vi "Conductance Background.vi"() -> ()   [LabVIEW 2021]
uses:
  <vilib>/Analysis/NI_AALPro.lvlib
  <vilib>/Analysis/polynomials.llb/1D Polynomial Evaluation (DBL).vi
panel:
  in  "Fit":bool
  in  "polynomial order":i32=2
  in  "BG polynom":dbl[](array[numeric])
  in  "BG2 length":i32
  in  "BG2 start":i32
  in  "BG1 length":i32
  in  "BG1 start":i32
  out "Background":cluster{dbl[], dbl[]}[](graph)
  out "Array - String":string[](array[string])
  out "Temperature vs scan number":cluster{dbl[], dbl[]}(graph)
  in  "Bacground correction":dbl
  in  "Temperature":string="Cryo-Con 32 (12) A"
  in  "Y":string="dIdV"
  in  "X":string="V"
  out "Scans":cluster{dbl[], dbl[]}[](graph)
  out "Scan temperatures":dbl[](array[numeric])
  in  "Scan indexes":i32[](array[numeric])=[1]
  in  "File Path":path=path "C:/Data/m010_072922.tdms"
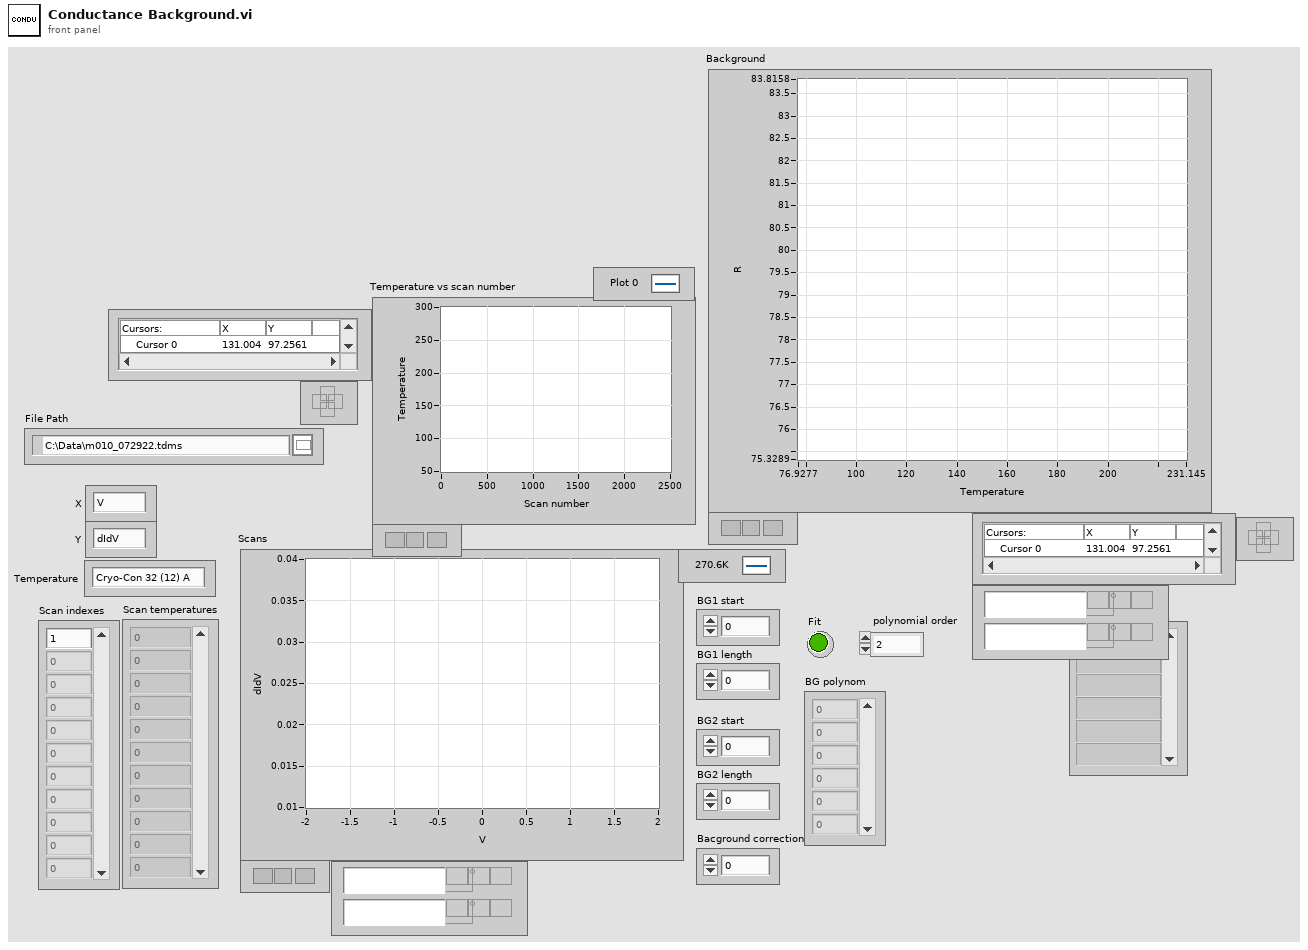
[diagram p1: front panel]
types:
  T1 = enum16{"open", "open or create", "create or replace", "create", "open (read-only)"}
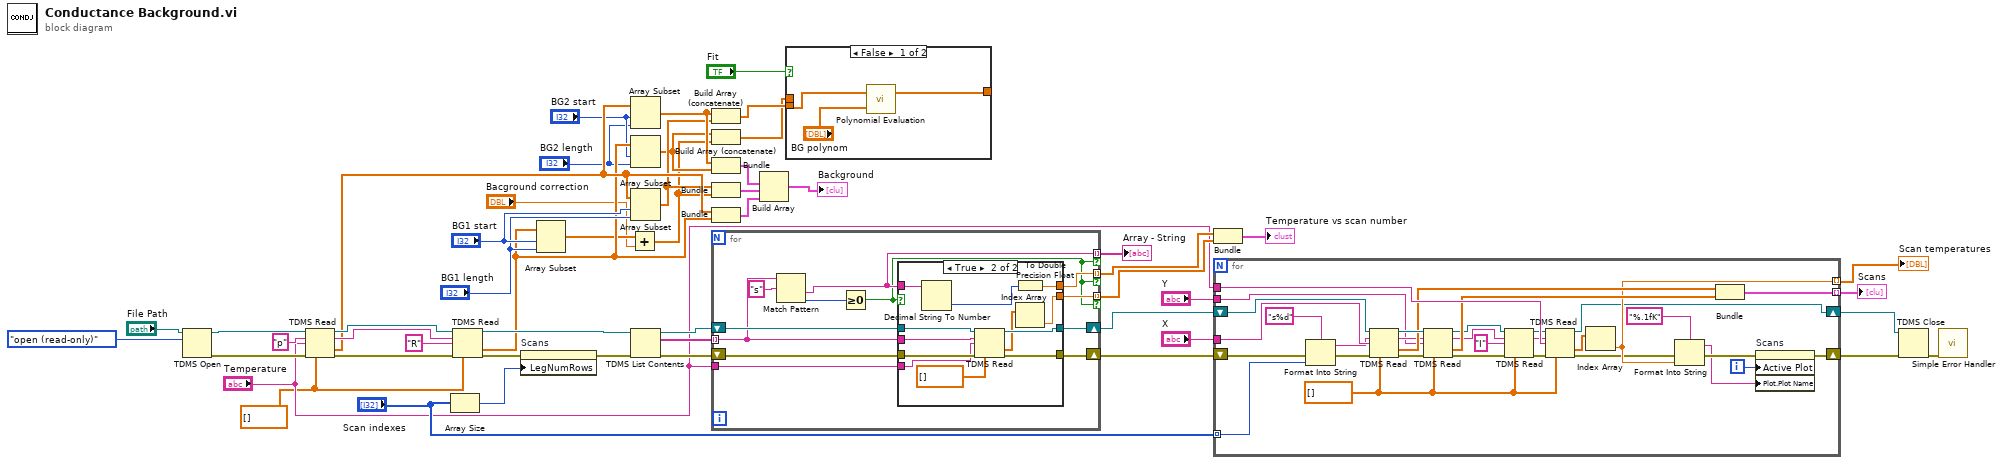
[diagram p0: block diagram]
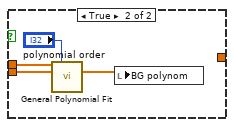
[diagram p2: hidden frame]
diagram:
  w20 = dbl[] []
  n1 = TDMS Open(10:T1."open (read-only)" ("operation (0:open)"), 11:"File Path") -> (0:w42:errorcluster, 3:w28:refnum<k34>)  [unwired: 5 in]
  n2 = TDMS Read(0:w28, 5:"p" ("group name in"), 7:"Temperature", 11:w42, 12:w20) -> (4:w26:refnum<k34>, 6:w23:string, 10:w14:dbl[], 15:w29:errorcluster)  [unwired: 3 in, 2 out]
  n3 = Array Size(array="Scan indexes") -> (size(s)=w43:i32)
  n4 = TDMS Read(0:w26, 5:w23, 7:"R" ("channel name(s) in"), 11:w29, 12:w20) -> (4:w25:refnum<k34>, 10:w13:dbl[], 15:w27:errorcluster)  [unwired: 3 in, 3 out]
  n5 = property on="Scans" class="XYGraph (strict)"(error in=w27, "LegNumRows"=w43) -> (error out=w36:errorcluster)  [unwired: 1 in, 1 out]
  n6 = Array Subset(array=w13, index="BG1 start", length="BG1 length") -> (w9:dbl[])
  n7 = Add(x=w9, y="Bacground correction") -> (x+y=w2:dbl[])
  n8 = Array Subset(array=w14, index="BG2 start", length="BG2 length") -> (w7:dbl[])
  n9 = Array Subset(array=w13, index="BG2 start", length="BG2 length") -> (w3:dbl[])
  n10 = Array Subset(array=w14, index="BG1 start", length="BG1 length") -> (w6:dbl[])
  n11 = TDMS List Contents(4:w36, 7:w25) -> (0:w38:errorcluster, 2:w39:string[], 3:w37:refnum<k34>)  [unwired: 1 in, 1 out]
  n12 = Build Array (concatenate)(w7, w6) -> (w5:dbl[])
  n13 = Build Array (concatenate)(w3, w2) -> (w4:dbl[])
  n14 = Bundle(w7, w3) -> (w12:cluster{dbl[], dbl[]})  [unwired: 1 in]
  n15 = Bundle(w6, w2) -> (w16:cluster{dbl[], dbl[]})  [unwired: 1 in]
  n16 = Bundle(w14, w13) -> (w15:cluster{dbl[], dbl[]})  [unwired: 1 in]
  n17 = for {
    tunnel: w39 -> [w59] mode=indexing
    tunnel: [w54] -> w33 mode=indexing if=w52
    shift-right: [w57] -> w34
    shift-left: w37 -> [w61]
    shift-right: [w56] -> w35
    shift-left: w38 -> [w60]
    tunnel: "Temperature" -> [w58]
    tunnel: [w55] -> w30 mode=indexing if=w52
    tunnel: [w53] -> w31 mode=indexing if=w52
    n18 = Match Pattern(string=w59, regular expression="s") -> (after substring=w54:string, offset past match=w62:i32)  [unwired: 1 in, 2 out]
    n19 = Greater Or Equal To 0?(x=w62) -> (x >= 0?=w52:bool)
    n20 = case shown="True" w52 {
      tunnel: w61 -> [w65 w77]
      tunnel: w60 -> [w64 w76]
      tunnel: w59 -> [_ w74]
      tunnel: w58 -> [_ w73]
      tunnel: [w65 w72] -> w57
      tunnel: [w64 w71] -> w56
      tunnel: [_ w69] -> w55
      tunnel: w54 -> [_ w68]
      tunnel: [_ w66] -> w53
      frame False {
      }
      frame True {
        n21 = Decimal String To Number(string=w68) -> (number=w67:i32)  [unwired: 2 in, 1 out]
        n22 = TDMS Read(0:w77, 5:w74, 7:w73, 11:w76, 12:dbl[] []) -> (4:w72:refnum<k34>, 10:w70:dbl[], 15:w71:errorcluster)  [unwired: 3 in, 3 out]
        n23 = To Double Precision Float(number=w67) -> (double precision float=w66:dbl)
        n24 = Index Array(array=w70) -> (element=w69:dbl)  [unwired: 1 in]
      }
    }
  }
  "Array - String" <- w33
  n25 = Build Array(w12, w16, w15) -> (→"Background":cluster{dbl[], dbl[]}[])  [unwired: 1 in]
  n26 = case shown="False" "Fit" {
    tunnel: w5 -> [w80 w84]
    tunnel: w4 -> [_ w83]
    tunnel: [w78 _] -> _
    frame False {
      n27 = call-poly <vilib>:"Polynomial Evaluation.vi"("P(x)"="BG polynom", "A"=w80) -> ("P(A)"=w78:dbl[])  [unwired: 1 out]
    }
    frame True {
      n28 = call <vilib>:"General Polynomial Fit.vi"("Y"=w83, "polynomial order"="polynomial order", "X"=w84) -> ("Polynomial Coefficients"=w81:dbl[])  [unwired: 9 in, 3 out]
      n29 = local write "BG polynom"(w81) -> ()
    }
  }
  n30 = Bundle(w31, w30) -> (→"Temperature vs scan number":cluster{dbl[], dbl[]})  [unwired: 1 in]
  n31 = for {
    tunnel: "Scan indexes" -> [w116] mode=indexing
    shift-right: [w103] -> w40
    shift-left: w35 -> [w114]
    tunnel: "Temperature" -> [w113]
    tunnel: [w100] -> w49 mode=indexing
    shift-right: [w86] -> w41
    shift-left: w34 -> [w97]
    tunnel: "X" -> [w106]
    tunnel: "Y" -> [w105]
    tunnel: [w104] -> w45 mode=indexing
    i -> [w101]
    w92 = dbl[] []
    n32 = Format Into String(format string="s%d", error in=w114, w116) -> (resulting string=w90:string, error out=w96:errorcluster)  [unwired: 1 in]
    n33 = TDMS Read(0:w97, 5:w90, 7:w106, 11:w96, 12:w92) -> (4:w110:refnum<k34>, 6:w107:string, 10:w109:dbl[], 15:w111:errorcluster)  [unwired: 3 in, 2 out]
    n34 = TDMS Read(0:w110, 5:w107, 7:w105, 11:w111, 12:w92) -> (4:w94:refnum<k34>, 6:w95:string, 10:w108:dbl[], 15:w93:errorcluster)  [unwired: 3 in, 2 out]
    n35 = TDMS Read(0:w94, 5:w95, 7:"I" ("channel name(s) in"), 11:w93, 12:w92) -> (4:w89:refnum<k34>, 6:w85:string, 15:w88:errorcluster)  [unwired: 3 in, 3 out]
    n36 = TDMS Read(0:w89, 5:w85, 7:w113, 11:w88, 12:w92) -> (4:w86:refnum<k34>, 10:w112:dbl[], 15:w87:errorcluster)  [unwired: 3 in, 3 out]
    n37 = Index Array(array=w112) -> (element=w100:dbl)  [unwired: 1 in]
    n38 = Format Into String(format string="%.1fK", error in=w87, w100) -> (resulting string=w98:string, error out=w102:errorcluster)  [unwired: 1 in]
    n39 = Bundle(w109, w108) -> (w104:cluster{dbl[], dbl[]})  [unwired: 1 in]
    n40 = property on="Scans" class="XYGraph (strict)"(error in=w102, "Active Plot"=w101, "Plot.Plot Name"=w98) -> (error out=w103:errorcluster)  [unwired: 1 in, 1 out]
  }
  "Scan temperatures" <- w49
  "Scans" <- w45
  n41 = TDMS Close(8:w40, 11:w41) -> (0:w48:errorcluster)  [unwired: 1 out]
  n42 = call <vilib>:"Simple Error Handler.vi"("error in (no error)"=w48) -> ()  [unwired: 4 in, 5 out]
